vi "Driver Joystick Outputs.vi"() -> (3 "Joy X":dbl, 4 "Joy Y":dbl, 5 "Robot Orientation":T1, 6 "Joy Twist":dbl)   [LabVIEW 2012]
uses:
  Controls/Robot Orientation.ctl
  <vilib>/Rock Robotics/WPI/Joystick/WPI_JoystickGetSetRefNum.vi
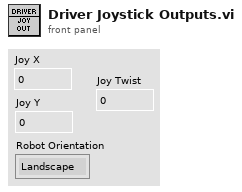
[diagram p1: front panel]
types:
  T1 = typedef "Robot Orientation.ctl" = enum16{"Landscape", "Portrait"}
  T2 = typedef "WPI_JoystickDevRef.ctl" = cluster{"Device":T3}
  T3 = typedef "WPI_JoystickDeviceEnum.ctl" = enum16{"USB 1", "USB 2", "USB 3", "USB 4", "Kinect 1", "Kinect 2"}
  T4 = typedef "WPI_JoystickButtonState.ctl" = cluster{"Button 1":bool, "Button 2":bool, "Button 3":bool, "Button 4":bool, "Button 5":bool, "Button 6":bool, "Button 7":bool, "Button 8":bool, "Button 9":bool, "Button 10":bool, "Button 11":bool, "Button 12":bool}
  T5 = cluster{"axis 1 (x)":dbl, "axis 2 (y)":dbl, "axis 3 (throttle)":dbl, "axis 4":dbl, "axis 5":dbl, "axis 6":dbl}
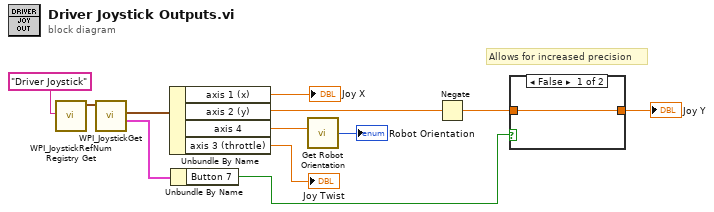
[diagram p0: block diagram]
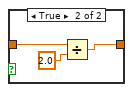
[diagram p2: hidden frame]
diagram:
  # "Allows for increased precision"
  n1 = call <vilib>:"WPI_JoystickRefNum Registry Get.vi"("refnum name"="Driver Joystick") -> ("JoystickDevRef"=w11:T2)  [unwired: 9 in, 1 out]
  n2 = call <vilib>:"WPI_JoystickGet.vi"("JoystickDevRef"=w11) -> ("Buttons"=w3:T4, "Axes"=w10:T5)  [unwired: 4 in, 1 out]
  n3 = Unbundle By Name(w10) -> ("axis 1 (x)"=→"Joy X":dbl, "axis 2 (y)"=w5:dbl, "axis 4"=w9:dbl, "axis 3 (throttle)"=→"Joy Twist":dbl)
  n4 = Unbundle By Name(w3) -> ("Button 7"=w1:bool)
  n5 = call "Get Robot Orientation.vi"("Throttle In"=w9) -> ("Robot Orientation Out"=→"Robot Orientation":T1)
  n6 = Negate(x=w5) -> (-x=w4:dbl)
  n7 = case shown="False" w1 {
    tunnel: w4 -> [w13 w16]
    tunnel: [w13 w15] -> w2
    frame False {
    }
    frame True {
      n8 = Divide(x=w16, y=2.0) -> (x/y=w15:dbl)
    }
  }
  "Joy Y" <- w2
